vi "Get Function List Path.vi"(8 "error in":errorcluster) -> (0 "error out":errorcluster, 3 "Functions List Path":path)   [LabVIEW 2016, in "function manager.lvclass"]
uses:
  function manager.lvclass
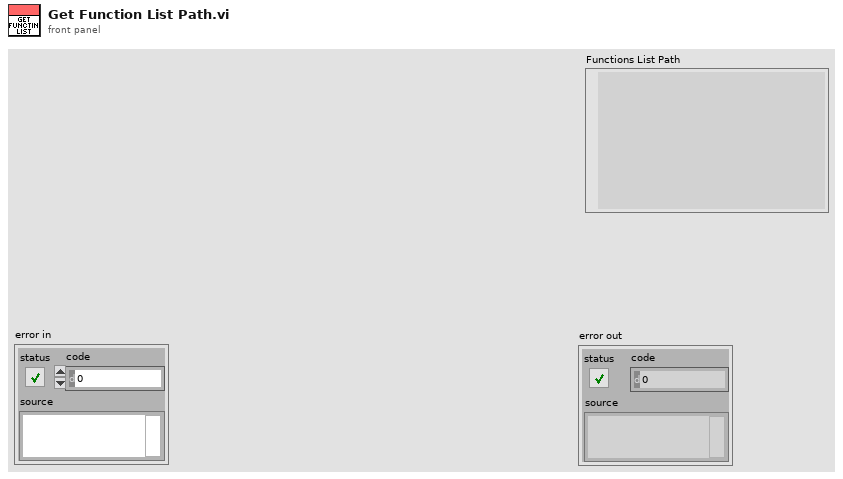
[diagram p1: front panel]
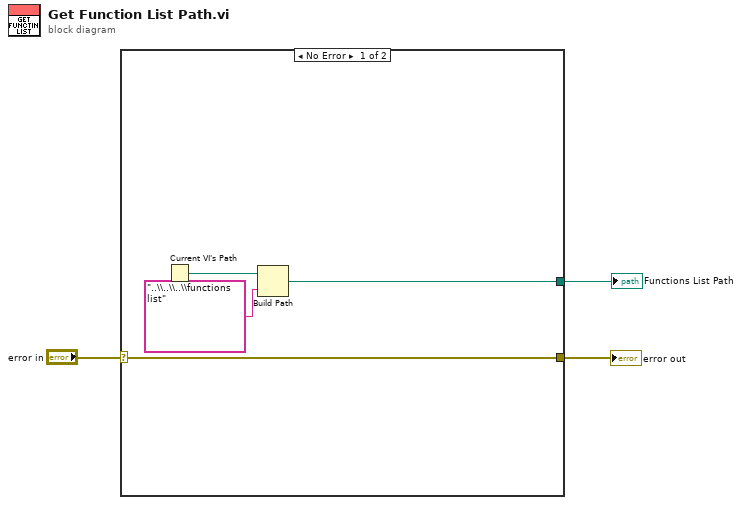
[diagram p0: block diagram]
diagram:
  n1 = case shown="No Error" "error in" {
    selector: "error in" -> [w7 w8]
    tunnel: [w7 w8] -> w2
    tunnel: [w4 _] -> w1
    frame No Error {
      n2 = Current VI's Path() -> (path=w6:path)
      n3 = Build Path(base path=w6, name or relative path="..\\..\\..\\functions list") -> (appended path=w4:path)
    }
    frame Error {
    }
  }
  "error out" <- w2
  "Functions List Path" <- w1
